vi "Variant to db String.vi"(10 "error in (no error)":errorcluster, 11 "Control Data":variant) -> (2 "error out":errorcluster, 3 "DB String":string, 5 "unsigned byte array":u8[](array[numeric]))   [LabVIEW 2017]
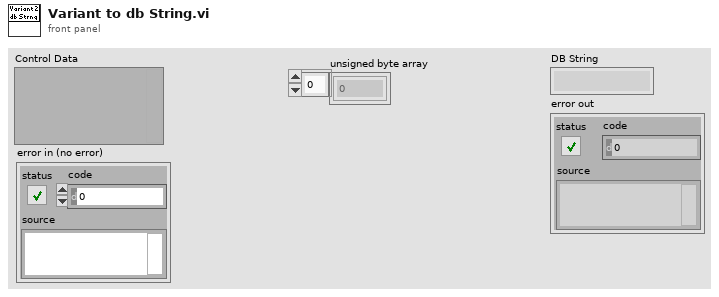
[diagram p1: front panel]
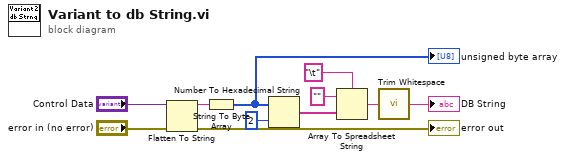
[diagram p0: block diagram]
diagram:
  n1 = Flatten To String(anything="Control Data", error in (no error)="error in (no error)") -> (data string=w6:string, error out=→"error out":errorcluster)  [unwired: 2 in, 1 out]
  n2 = String To Byte Array(string=w6) -> (unsigned byte array=w11:u8[])
  "unsigned byte array" <- w11
  n3 = Number To Hexadecimal String(1:i16 2 ("width (-)"), 2:w11) -> (0:w9:string[])
  n4 = Array To Spreadsheet String(delimiter (Tab)="\t", array=w9, 3:"" ("format string")) -> (spreadsheet string=w3:string)
  n5 = call <vilib>:"Trim Whitespace.vi"("string"=w3) -> ("trimmed string"=→"DB String":string)  [unwired: 1 in]
